vi "Low-Pass_Filter.vi"(6 "Ts":dbl=1000.0 min=50.0 max=20000.0 format="%#_13g", 7 "Tf":dbl=1000.0 min=50.0 max=20000.0 format="%#_13g", 9 "Input":dbl=1000.0 min=50.0 max=20000.0 format="%#_13g") -> (2 "Filter Output":dbl=1000.0 min=50.0 max=20000.0 format="%#_13g")   [LabVIEW 2019]
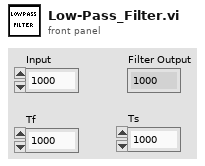
[diagram p1: front panel]
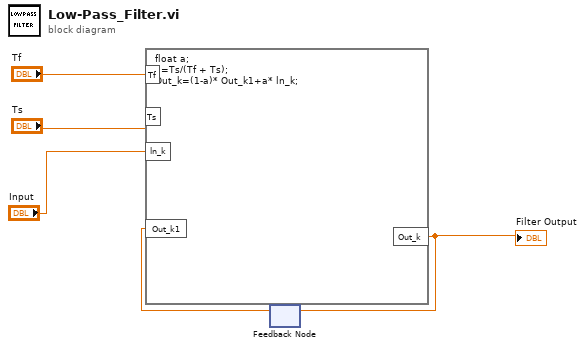
[diagram p0: block diagram]
diagram:
  n1 = feedback #1() -> (w5:dbl)  [unwired: 1 in]
  n2 = formula code="float a;\na=Ts/(Tf + Ts);\nOut_k=(1-a)* Out_k1+a* ln_k;"("Tf"="Tf", "Ts"="Ts", "ln_k"="Input", "Out_k1"=w5) -> ("Out_k"=w4:dbl)
  "Filter Output" <- w4
  n3 = feedback-in #1(w4) -> ()
